vi "testRemoveOutOfRangeHigh.vi"(8 "error in (no error)":errorcluster, 11 "TestCase in":refnum<class "ListImp_Common.lvclass">) -> (0 "error out":errorcluster, 3 "TestCase out":refnum<class "ListImp_Common.lvclass">)   [LabVIEW 2013, in "ListImp_Common.lvclass"]
uses:
  ListImp_Common.lvclass
  ListImp_Common.lvclass/ListImp_Common.ctl
  source/LapDog.Collections.Lists/ListImp/ListImp.lvclass
  <vilib>/addons/_JKI Toolkits/VI Tester/TestCase.llb/TestCase.lvclass
  UnitTestComparisons/UnitTestComparisons.lvlib
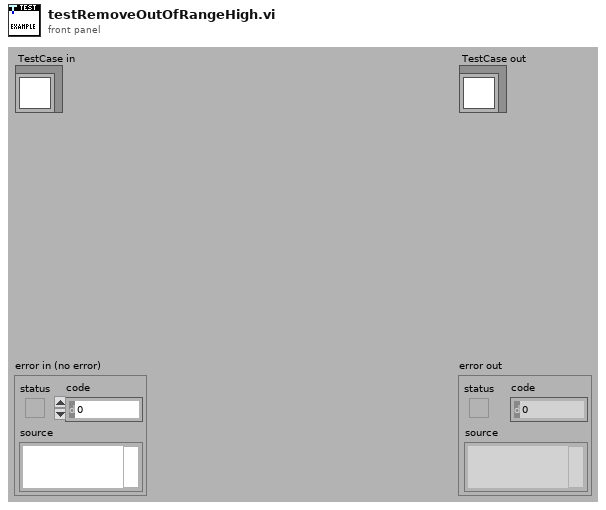
[diagram p1: front panel]
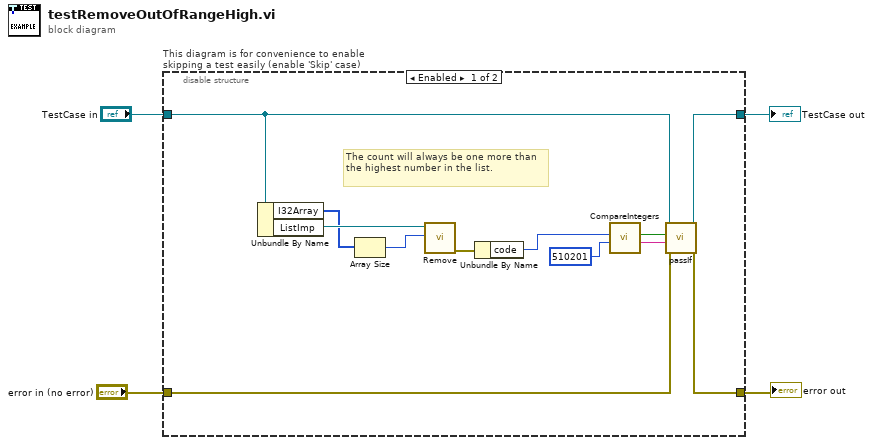
[diagram p0: block diagram]
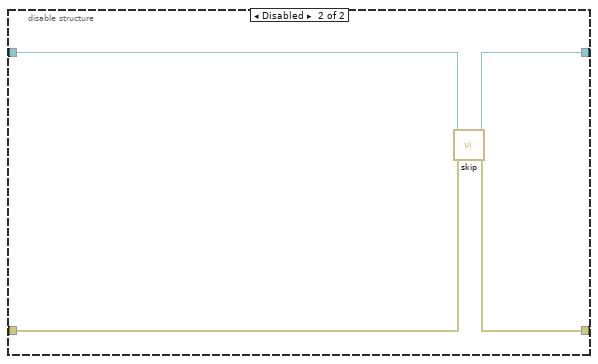
[diagram p2: hidden frame]
diagram:
  n1 = disable-structure "This diagram is for convenience to enable skipping a test easily (enable 'Skip' case)" shown="Enabled" {
    disable-tunnel: "TestCase in" -> [w13 w20]
    disable-tunnel: [w16 w18] -> w1
    disable-tunnel: [w15 w19] -> w3
    disable-tunnel: "error in (no error)" -> [w14 w17]
    frame Enabled {
      # "The count will always be one more than the highest number in the list."
      n2 = Unbundle By Name(w13) -> ("I32Array"=w6:i32[], "ListImp"=w7:refnum<class "ListImp.lvclass">)
      n3 = Array Size(array=w6) -> (size(s)=w5:i32)
      n4 = call-dynamic "Remove.vi"("Index"=w5, "ListImp in"=w7) -> ("error out"=w9:errorcluster)  [unwired: 7 in, 2 out]
      n5 = Unbundle By Name(w9) -> ("code"=w8:i32)
      n6 = call "CompareIntegers.vi"("Expected Value"=510201, "Actual Value"=w8) -> ("Message"=w11:string, "Equal?"=w12:bool)  [unwired: 8 in]
      n7 = call-dynamic "passIf.vi"("error in (no error)"=w14, "message (\"\")"=w11, "pass"=w12, "TestCase in"=w13) -> ("error out"=w15:errorcluster, "TestCase out"=w16:refnum<class "ListImp_Common.lvclass">)  [unwired: 6 in]
    }
    frame Disabled {
      # "skip test result while test is under development"
      n8 = call <vilib>:"skip.vi"("error in (no error)"=w17, "TestCase in"=w20) -> ("error out"=w19:errorcluster, "TestCase out"=w18:refnum<class "ListImp_Common.lvclass">)  [unwired: 8 in]
    }
  }
  "error out" <- w3
  "TestCase out" <- w1
